vi "Field Draw Ball.vi"(3 "Project":T2=enum."VSS", 4 "Draw Targets?":T3, 5 "KeeperPlay":T1=enum."NormalGame", 6 "Lado":enum16{"Esquerdo", "Direito"}(ring), 7 "Referee":refnum<class "Referee.lvclass">=refnum, 8 "picture in":picture, 9 "Offset":T4, 10 "Scale mm/pixel":dbl, 11 "BallRef":refnum<class "Ball.lvclass">=refnum) -> (0 "picture out":picture)   [LabVIEW 2022 SP3]
uses:
  Ball_class/Ball.lvclass
  <vilib>/Analysis/NI_AALPro.lvlib
  Referee_class/Referee.lvclass
  <vilib>/Analysis/coordinate.llb/2D Cartesian Coordinate Rotation (Scalar).vi
  <vilib>/Utility/miscctls.llb/LVBoundsTypeDef.ctl
  DrawTargets.ctl
  Project.ctl
  Team_class/KeeperPlay.ctl
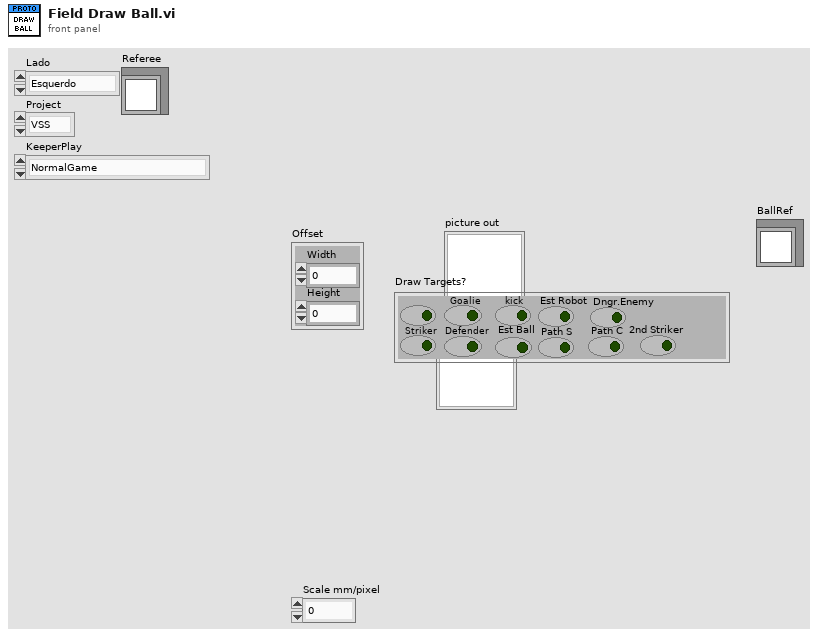
[diagram p1: front panel]
types:
  T1 = typedef "KeeperPlay.ctl" = enum16{"SimpleBallPlacementAlly", "BallPlacementAlly", "BallPlacementEnemy", "ZigZag", "Goto", "NormalGame", "KeeperPlay", "Halt", "Timeout", "PenaltyEnemy", "TestPlay"}
  T2 = typedef "Project.ctl" = enum16{"SSL", "VSS"}
  T3 = typedef "DrawTargets.ctl" = cluster{"Attacker":bool, "Striker":bool, "Goalie":bool, "Defender":bool, "kick":bool, "Est Ball":bool, "Est Robot":bool, "Path S":bool, "Path C":bool, "Dngr.Enemy":bool, "2nd Striker":bool}
  T4 = typedef "LVBoundsTypeDef.ctl" = cluster{"Width":u32, "Height":u32}
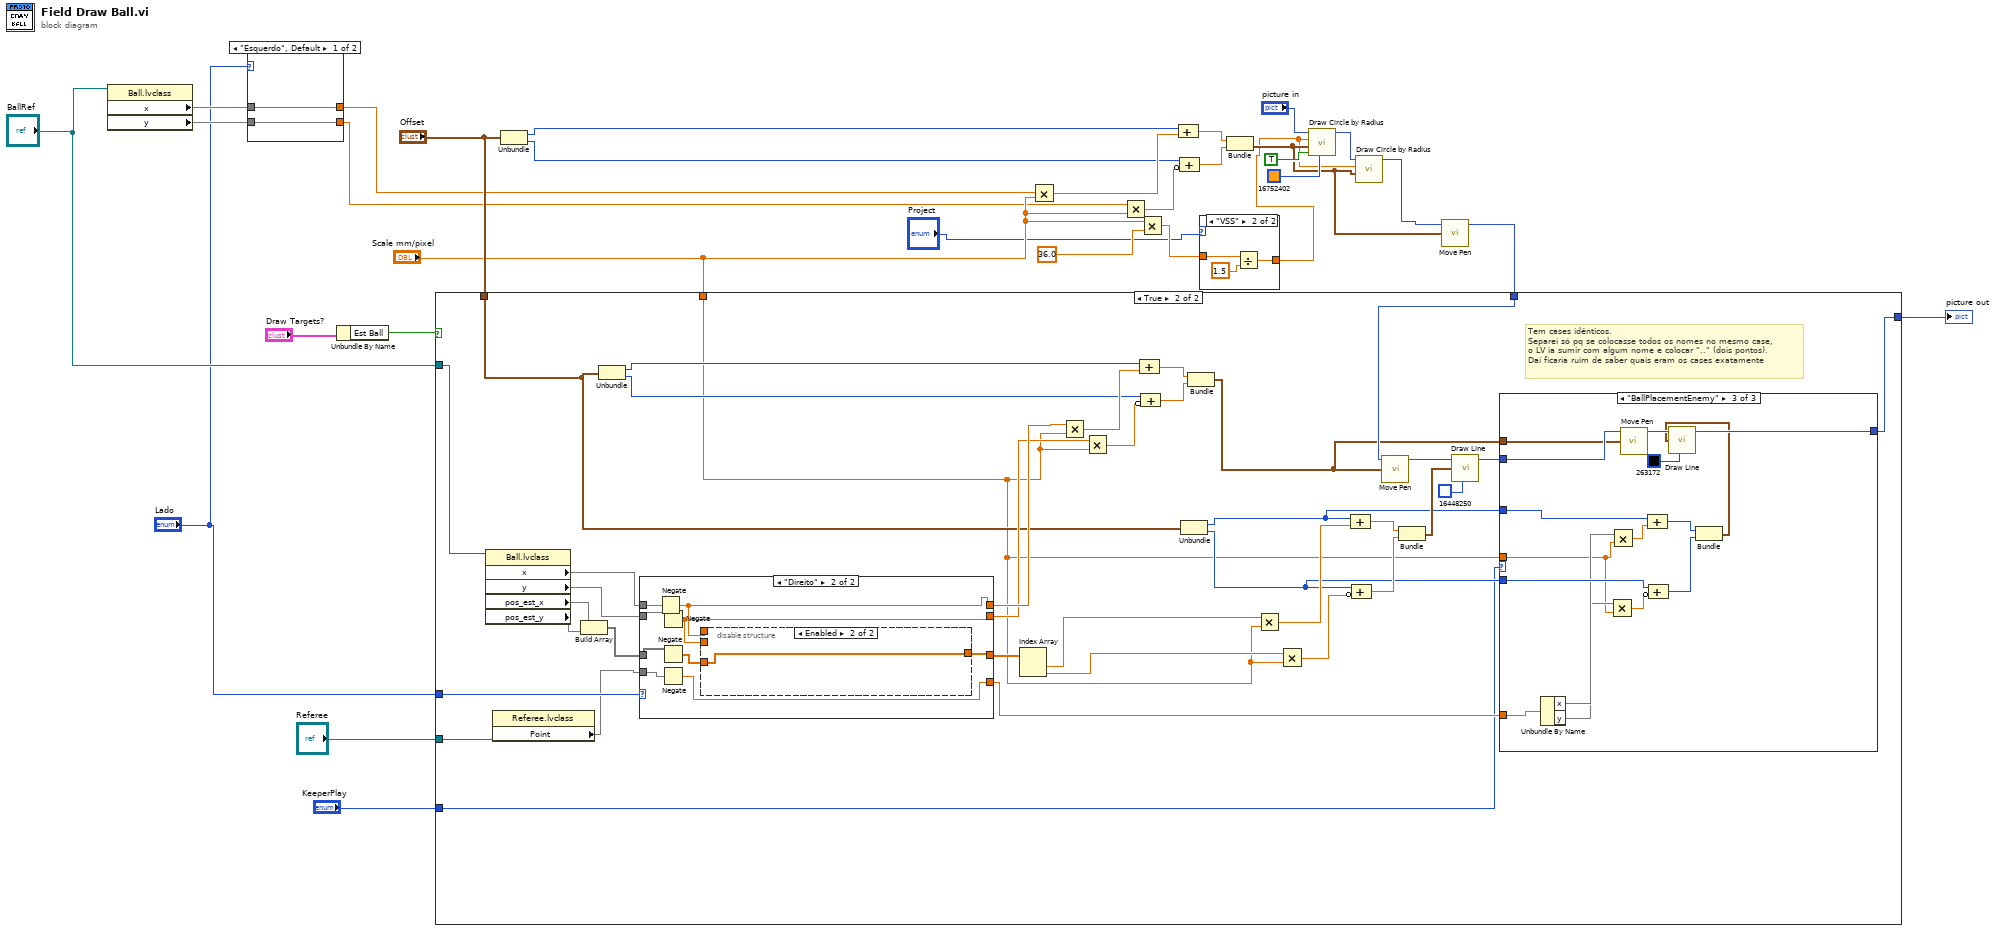
[diagram p0: block diagram]
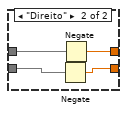
[diagram p3: hidden frame]
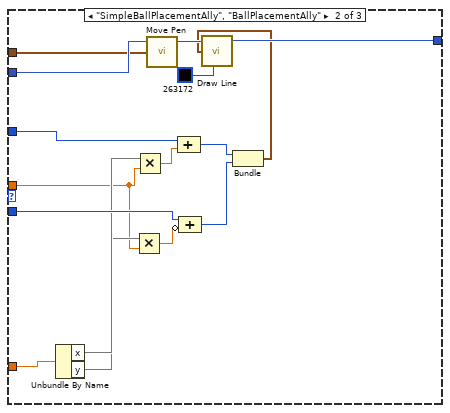
[diagram p6: hidden frame]
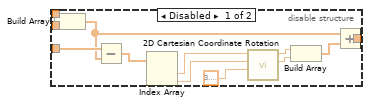
[diagram p8: hidden frame]
diagram:
  n1 = property class="Ball.lvclass"(reference="BallRef") -> ("x"=w8, "y"=w7)  [unwired: 1 in, 2 out]
  n2 = case shown="\"Esquerdo\", Default" "Lado" {
    tunnel: [w32 w36] -> w10
    tunnel: w8 -> [w32 w33]
    tunnel: [w31 w34] -> w9
    tunnel: w7 -> [w31 w35]
    frame "Esquerdo", Default {
    }
    frame "Direito" {
      n3 = Negate(x=w35) -> (-x=w34:dbl)
      n4 = Negate(x=w33) -> (-x=w36:dbl)
    }
  }
  n5 = Unbundle By Name("Draw Targets?") -> ("Est Ball"=w12:bool)
  n6 = Unbundle("Offset") -> ("Width"=w27:u32, "Height"=w24:u32)
  n7 = Multiply(x=w10, y="Scale mm/pixel") -> (x*y=w26:dbl)
  n8 = Multiply(x=w9, y="Scale mm/pixel") -> (x*y=w23:dbl)
  n9 = Multiply(x="Scale mm/pixel", y=sgl 36.0 ("radius")) -> (x*y=w5:dbl)
  n10 = Compound Arithmetic op=ADD(w27, w26) -> (w25:dbl)
  n11 = Compound Arithmetic op=ADD(w24, invert w23) -> (w22:dbl)
  n12 = case shown="\"VSS\"" "Project" {
    tunnel: w5 -> [w37 w40]
    tunnel: [w37 w38] -> w4
    frame "SSL", Default {
    }
    frame "VSS" {
      n13 = Divide(x=w40, y=1.5) -> (x/y=w38:dbl)
    }
  }
  n14 = Bundle(w25, w22) -> (w16:cluster{dbl, dbl})  [unwired: 1 in]
  n15 = call <vilib>:"Draw Circle by Radius.vi"("color(black)"=u32 16752402, "fill?(F)"=TRUE, "pixel center"=w16, "radius"=w4, "picture"="picture in") -> ("new picture"=w20:picture)  [unwired: 6 in]
  n16 = call <vilib>:"Draw Circle by Radius.vi"("pixel center"=w16, "radius"=w4, "picture"=w20) -> ("new picture"=w17:picture)  [unwired: 8 in]
  n17 = call <vilib>:"Move Pen.vi"("new position"=w16, "picture"=w17) -> ("new picture"=w18:picture)  [unwired: 3 in]
  n18 = case shown="True" w12 {
    tunnel: [w41 w47] -> w19
    tunnel: w18 -> [w41 w53]
    tunnel: "Offset" -> [_ w55]
    tunnel: "Scale mm/pixel" -> [_ w45]
    tunnel: "BallRef" -> [_ w54]
    tunnel: "Lado" -> [_ w52]
    tunnel: "Referee" -> [_ w49]
    tunnel: "KeeperPlay" -> [_ w42]
    frame False {
    }
    frame True {
      # "Tem cases idênticos.\nSeparei só pq se colocasse todos os nomes no mesmo case,\no LV ia sumir com algum nome e colocar \"..\" (dois pontos).\nDaí ficaria ruim de saber quais eram os cases exatamente"
      n19 = property class="Ball.lvclass"(reference=w54) -> ("x"=w56, "y"=w57, "pos_est_x"=w60, "pos_est_y"=w59)  [unwired: 1 in, 2 out]
      n20 = property class="Referee.lvclass"(reference=w49) -> ("Point"=w44)  [unwired: 1 in, 2 out]
      n21 = Build Array(w60, w59) -> (w58:void[])
      n22 = Unbundle(w55) -> ("Width"=w78:u32, "Height"=w75:u32)
      n23 = case shown="\"Direito\"" w52 {
        tunnel: [w115 w121] -> w63
        tunnel: w56 -> [w115 w124]
        tunnel: [w114 w120] -> w62
        tunnel: w57 -> [w114 w123]
        tunnel: [w113 w119] -> w61
        tunnel: w58 -> [w113 w122]
        tunnel: w44 -> [w112 w116]
        tunnel: [w112 w117] -> w43
        frame "Esquerdo", Default {
        }
        frame "Direito" {
          n24 = Negate(x=w124) -> (-x=w121:dbl)
          n25 = Negate(x=w123) -> (-x=w120:dbl)
          n26 = Negate(x=w122) -> (-x=w118:dbl[])
          n27 = Negate(x=w116) -> (-x=w117:dbl)
          n28 = disable-structure shown="Enabled" {
            disable-tunnel: w121 -> [w131 _]
            disable-tunnel: w120 -> [w130 _]
            disable-tunnel: w118 -> [w129 w137]
            disable-tunnel: [w127 w137] -> w119
            frame Disabled {
              n29 = Build Array(w131, w130) -> (w125:dbl[])
              n30 = Subtract(x=w129, y=w125) -> (x-y=w128:dbl[])
              n31 = Index Array(array=w128) -> (element #1=w136:dbl, element #2=w135:dbl)  [unwired: 2 in]
              n32 = call-poly <vilib>:"2D Cartesian Coordinate Rotation.vi"("theta"=3.141592653589793, "y"=w135, "x"=w136) -> ("y out"=w133:dbl, "x out"=w134:dbl)  [unwired: 6 in, 1 out]
              n33 = Build Array(w134, w133) -> (w126:dbl[])
              n34 = Add(x=w125, y=w126) -> (x+y=w127:dbl[])
            }
            frame Enabled {
            }
          }
        }
      }
      n35 = Index Array(array=w61) -> (element #1=w66:dbl, element #2=w65:dbl)  [unwired: 2 in]
      n36 = Multiply(x=w63, y=w45) -> (x*y=w77:dbl)
      n37 = Multiply(x=w62, y=w45) -> (x*y=w74:dbl)
      n38 = Compound Arithmetic op=ADD(w78, w77) -> (w76:dbl)
      n39 = Compound Arithmetic op=ADD(w75, invert w74) -> (w73:dbl)
      n40 = Unbundle(w55) -> ("Width"=w51:u32, "Height"=w50:u32)
      n41 = Bundle(w76, w73) -> (w46:cluster{dbl, dbl})  [unwired: 1 in]
      n42 = Multiply(x=w66, y=w45) -> (x*y=w68:dbl)
      n43 = Multiply(x=w65, y=w45) -> (x*y=w67:dbl)
      n44 = Compound Arithmetic op=ADD(w51, w68) -> (w71:dbl)
      n45 = Compound Arithmetic op=ADD(w50, invert w67) -> (w70:dbl)
      n46 = call <vilib>:"Move Pen.vi"("new position"=w46, "picture"=w53) -> ("new picture"=w72:picture)  [unwired: 3 in]
      n47 = Bundle(w71, w70) -> (w69:cluster{dbl, dbl})  [unwired: 1 in]
      n48 = call <vilib>:"Draw Line.vi"("picture"=w72, "end point"=w69, "color(black)"=u32 16448250) -> ("new picture"=w48:picture)  [unwired: 6 in]
      n49 = case shown="\"BallPlacementEnemy\"" w42 {
        tunnel: w51 -> [_ w93 w109]
        tunnel: w50 -> [_ w92 w108]
        tunnel: w48 -> [w79 w89 w105]
        tunnel: [w79 w88 w104] -> w47
        tunnel: w46 -> [_ w87 w103]
        tunnel: w45 -> [_ w83 w99]
        tunnel: w43 -> [_ w80 w96]
        frame Default {
        }
        frame "SimpleBallPlacementAlly", "BallPlacementAlly" {
          n50 = Unbundle By Name(w80) -> ("x"=w85, "y"=w84)
          n51 = Multiply(x=w84, y=w83) -> (x*y=w81:dbl)
          n52 = Multiply(x=w85, y=w83) -> (x*y=w82:dbl)
          n53 = call <vilib>:"Move Pen.vi"("new position"=w87, "picture"=w89) -> ("new picture"=w90:picture)  [unwired: 3 in]
          n54 = Compound Arithmetic op=ADD(w93, w82) -> (w95:u32)
          n55 = Compound Arithmetic op=ADD(w92, invert w81) -> (w94:u32)
          n56 = Bundle(w95, w94) -> (w86:cluster{u32, u32})  [unwired: 1 in]
          n57 = call <vilib>:"Draw Line.vi"("picture"=w90, "end point"=w86, "color(black)"=u32 263172) -> ("new picture"=w88:picture)  [unwired: 6 in]
        }
        frame "BallPlacementEnemy" {
          n58 = Unbundle By Name(w96) -> ("x"=w101, "y"=w100)
          n59 = Multiply(x=w100, y=w99) -> (x*y=w97:dbl)
          n60 = Multiply(x=w101, y=w99) -> (x*y=w98:dbl)
          n61 = call <vilib>:"Move Pen.vi"("new position"=w103, "picture"=w105) -> ("new picture"=w106:picture)  [unwired: 3 in]
          n62 = Compound Arithmetic op=ADD(w109, w98) -> (w111:u32)
          n63 = Compound Arithmetic op=ADD(w108, invert w97) -> (w110:u32)
          n64 = Bundle(w111, w110) -> (w102:cluster{u32, u32})  [unwired: 1 in]
          n65 = call <vilib>:"Draw Line.vi"("picture"=w106, "end point"=w102, "color(black)"=u32 263172) -> ("new picture"=w104:picture)  [unwired: 6 in]
        }
      }
    }
  }
  "picture out" <- w19
